vi "Get ParameterName.vi"(8 "Error In":errorcluster, 11 "reference in":refnum<class "OD Entry.lvclass">) -> (0 "Error Out":errorcluster, 2 "ParameterName":string, 3 "reference out":refnum<class "OD Entry.lvclass">)   [LabVIEW 2024, in "EDS.lvlib" / "OD Entry.lvclass"]
uses:
  OD Entry.lvclass
  OD Entry.lvclass/OD Entry.ctl
  Object Type/Object Type Base.lvclass
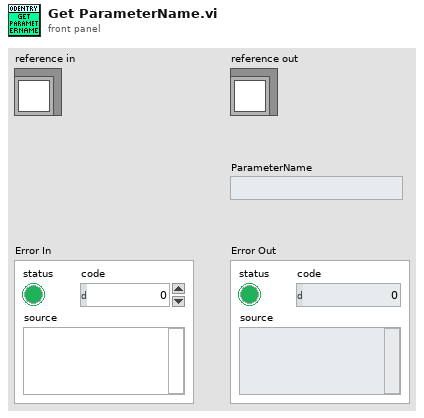
[diagram p1: front panel]
types:
  T1 = typedef "EDS.lvlib/OD Entry.lvclass/ObjectAttributes.ctl" = cluster{"Index":u16, "ObjectType":refnum<class "Object Type Base.lvclass">, "Denotation":string, "Count":u8, "ObjExtend":u8, "PDOtype":T2, "Label":string, "Description":string, "Sub-Entries":map{u8, refnum<class "OD Sub-Entry.lvclass">}}
  T2 = typedef "EDS.lvlib/PDO Mapping Type.ctl" = enum16{"NO", "OPTIONAL", "RPDO", "TPDO", "DEFAULT"}
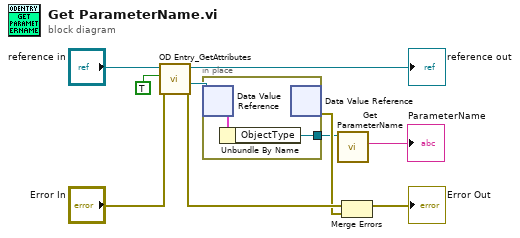
[diagram p0: block diagram]
diagram:
  n1 = call "OD Entry_GetAttributes.vi"("Error In"="Error In", "OnlyGetDvrReference(False)"=TRUE, "reference in"="reference in") -> ("Error Out"=w5:errorcluster, "DataRef"=w2:refnum<data-value>, "reference out"=→"reference out":refnum<class "OD Entry.lvclass">)  [unwired: 5 in, 1 out]
  n2 = in-place {
    in-place-border: [w12] -> w1
    n3 = in-place-dvr #1(w2) -> (w11:T1)  [unwired: 1 out]
    n4 = Unbundle By Name(w11) -> ("ObjectType"=w12:refnum<class "Object Type Base.lvclass">)
    n5 = in-place-dvr #1() -> (w4:errorcluster)  [unwired: 1 in, 1 out]
  }
  n6 = call "Get ParameterName.vi"("Object Type in"=w1) -> ("ParameterName"=→"ParameterName":string)  [unwired: 8 in, 2 out]
  n7 = Merge Errors(w5, w4) -> (→"Error Out":errorcluster)
